vi "Base Error Offset.vi"() -> (3 "base error offset":i32)   [LabVIEW 2021, in "DSF Core.lvlib" / "Component Loader.lvclass"]
uses:
  Component Loader.lvclass
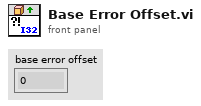
[diagram p1: front panel]
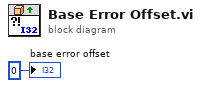
[diagram p0: block diagram]
diagram:
  "base error offset" <- 0 ("base error code")
